vi "Normalize Coordinates.vi"(9 "Camera Type":T1, 10 "Targets":T4(array[cluster]), 11 "Image in":T5) -> (1 "Camera view angles":dbl[](array[numeric])=[51.7, 49.4, 64.0, 52.0, 41.0], 2 "Found Targets":T2(array[cluster]) {"Normalized Rect"."Numeric 5" format="%#_2g"; "Normalized Rect"."Numeric 3" format="%#_2g"; "Normalized Rect"."Numeric 2" format="%#_2g"; "Normalized Rect"."Numeric" format="%#_2g"}, 3 "Sorted Scores":T3(array[cluster]) {"Moment Factor" format="%#_3g"; "L" format="%#_3g"; "Area to CH" format="%#_3g"; "X" format="%#_3g"; "Y" format="%#_3g"})   [LabVIEW 2015]
doc: "Normalize the rectangle and center so that they range from -1 to 1, left to right and bottom to top. This helps with producing joystick coordinates for driving the robot and makes the code better at handling resolution changes of the camera."
uses:
  <vilib>/vision/Image Controls.llb/IMAQ Image.ctl
  Camera Types.ctl
panel:
  # "Aspect Ratio"
  # "Density Profile"
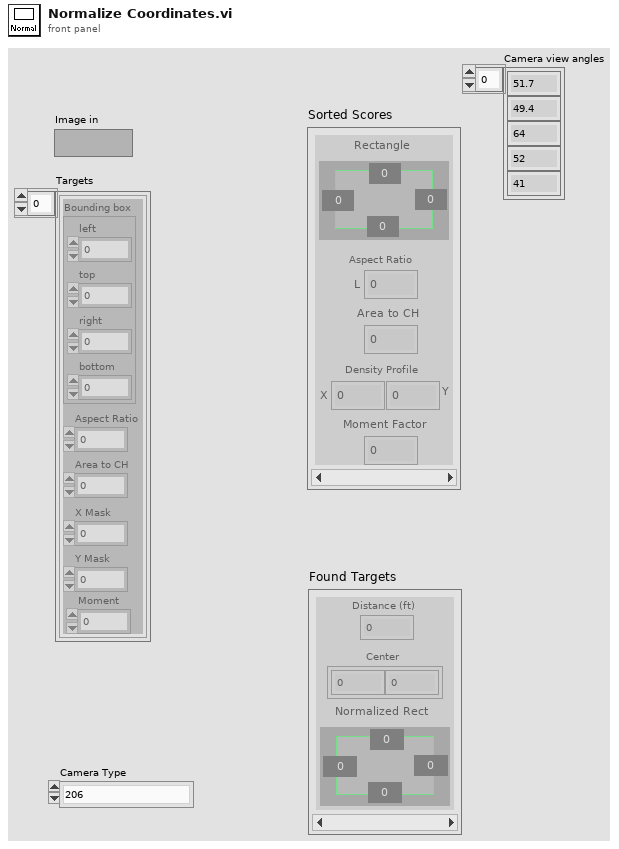
[diagram p1: front panel]
types:
  T1 = typedef "Camera Types.ctl" = enum16{"206", "1011", "1013", "MS HD3000 square", "MS HD3000 640x480"}
  T2 = cluster{"Distance (ft)":dbl, "Center":cluster{dbl, dbl}, "Normalized Rect":cluster{"Numeric":dbl, "Numeric 2":dbl, "Numeric 3":dbl, "Numeric 5":dbl}}[]
  T3 = cluster{"Rectangle":cluster{"Numeric":dbl, "Numeric 2":dbl, "Numeric 3":dbl, "Numeric 5":dbl}, "L":dbl, "Area to CH":dbl, "X":dbl, "Y":dbl, "Moment Factor":dbl}[]
  T4 = cluster{"Bounding box":cluster{"left":dbl, "top":dbl, "right":dbl, "bottom":dbl}, "Aspect Ratio":dbl, "Area to CH":dbl, "X Mask":dbl, "Y Mask":dbl, "Moment":dbl}[]
  T5 = typedef "IMAQ Image.ctl" = refnum<image>
  T6 = cluster{"left":dbl, "top":dbl, "right":dbl, "bottom":dbl}
  T7 = cluster{"X Resolution":i32, i32, "X Resolution":i32, i32}
  T8 = cluster{"Distance (ft)":dbl, cluster{dbl, dbl}, cluster{dbl, dbl, dbl, dbl}}
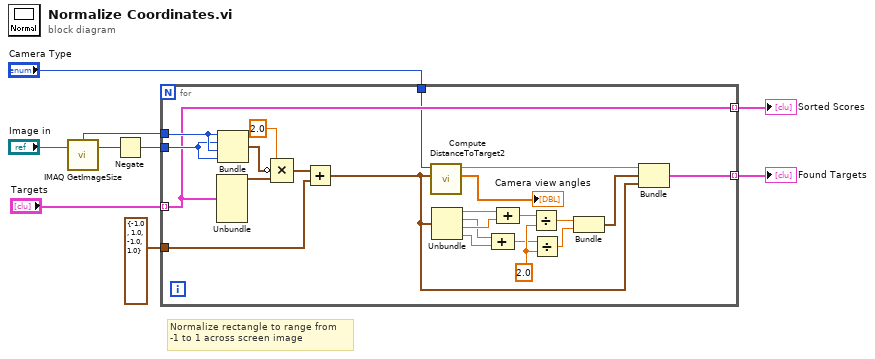
[diagram p0: block diagram]
diagram:
  # "Normalize rectangle to range from\n-1 to 1 across screen image"
  n1 = call "IMAQ GetImageSize"("Image"="Image in") -> ("Y Resolution"=w7:i32, "X Resolution"=w8:i32)  [unwired: 3 in, 1 out]
  n2 = Negate(x=w7) -> (-x=w9:i32)
  n3 = for {
    tunnel: "Targets" -> [w13] mode=indexing
    tunnel: w9 -> [w31]
    tunnel: w8 -> [w32]
    tunnel: [w17] -> w4 mode=indexing
    tunnel: [w13] -> w1 mode=indexing
    tunnel: cluster{dbl, dbl, dbl, dbl} {-1.0, 1.0, -1.0, 1.0} ("y") -> [w12]
    tunnel: "Camera Type" -> [w11]
    w22 = 2.0
    n4 = Unbundle(w13) -> ("Bounding box"=w29:T6)  [unwired: 5 out]
    n5 = Bundle("X Resolution"=w32, w31, "X Resolution"=w32, w31) -> (w30:T7)  [unwired: 1 in]
    n6 = Compound Arithmetic op=MULTIPLY(2.0, invert w30, w29) -> (w28:cluster{dbl, dbl, dbl, dbl})
    n7 = Add(x=w28, y=w12) -> (x+y=w16:cluster{dbl, dbl, dbl, dbl})
    n8 = call "Compute DistanceToTarget2.vi"("Normalized Rect"=w16, "Camera Type"=w11) -> ("Camera view angles"=→"Camera view angles":dbl[], "Distance (ft)"=w15:dbl)  [unwired: 8 in]
    n9 = Unbundle(w16) -> (w26:dbl, w23:dbl, w25:dbl, w24:dbl)
    n10 = Compound Arithmetic op=ADD(w23, w24) -> (w20:dbl)
    n11 = Compound Arithmetic op=ADD(w26, w25) -> (w21:dbl)
    n12 = Divide(x=w21, y=w22) -> (x/y=w19:dbl)
    n13 = Divide(x=w20, y=w22) -> (x/y=w18:dbl)
    n14 = Bundle(w19, w18) -> (w14:cluster{dbl, dbl})  [unwired: 1 in]
    n15 = Bundle("Distance (ft)"=w15, w14, w16) -> (w17:T8)  [unwired: 1 in]
  }
  "Sorted Scores" <- w1
  "Found Targets" <- w4
